vi "fix custom device xml.vi"(8 "error in (no error)":errorcluster, 10 "new xml path":path, 11 "CD name":string) -> (0 "error out":errorcluster)   [LabVIEW 2014, in "CD model script.lvlib"]
uses:
  CD model script.lvlib
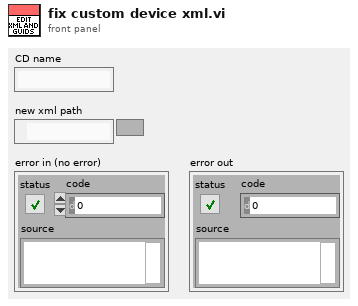
[diagram p1: front panel]
types:
  T1 = enum16{"open", "replace", "create", "open or create", "replace or create", "replace or create with confirmation"}
  T2 = typedef "CD model script.lvlib/CD Wizard - Extra Page Name and GUID.ctl" = cluster{"Page Name":string, "Page GUID":string}
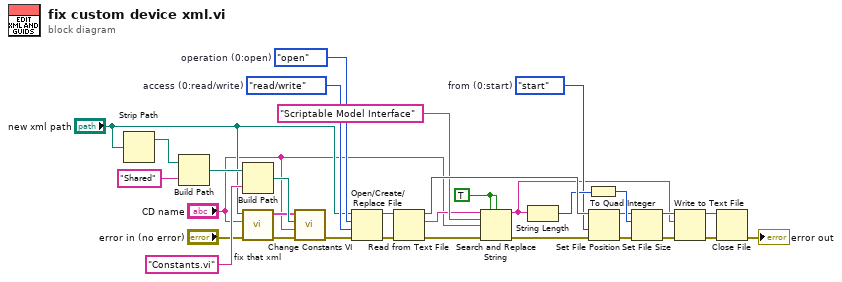
[diagram p0: block diagram]
diagram:
  w28 = enum16{"start", "end", "current"}."start"  # from (0:start)
  w21 = TRUE ("replace all? (F)")
  w17 = T1."open"  # operation (0:open)
  w16 = enum16{"read/write", "read-only", "write-only"}."read/write"  # access (0:read/write)
  n1 = Strip Path(path="new xml path") -> (stripped path=w11:path)  [unwired: 1 out]
  n2 = Build Path(base path=w11, name or relative path="Shared") -> (appended path=w10:path)
  n3 = Build Path(base path=w10, name or relative path="Constants.vi") -> (appended path=w7:path)
  n4 = call "fix that xml.vi"("error in (no error)"="error in (no error)", "nw CD name"="CD name", "Path"="new xml path") -> ("error out"=w12:errorcluster, "Extra Pages"=w6:T2[])  [unwired: 7 in]
  n5 = call "Change Constants VI.vi"("error in (no error)"=w12, "new cd name"="CD name", "Constants.vi path"=w7, "Extra Pages"=w6) -> ("error out"=w5:errorcluster)  [unwired: 7 in]
  n6 = Open/Create/Replace File(file path (use dialog)="new xml path", error in=w5, operation (0:open)=w17, access (0:read/write)=w16) -> (refnum out=w14:refnum<file>, error out=w15:errorcluster)  [unwired: 3 out]
  n7 = Read from Text File(file (use dialog)=w14, error in=w15) -> (refnum out=w31:refnum<file>, text=w18:string, error out=w19:errorcluster)  [unwired: 3 out]
  n8 = Search and Replace String(replace all?=w21, case sensitive?=w21, input string=w18, search string="Scriptable Model Interface", replace string="CD name", error in=w19) -> (result string=w13:string, error out=w32:errorcluster)  [unwired: 2 in, 2 out]
  n9 = String Length(string=w13) -> (length=w29:i32)
  n10 = To Quad Integer(1:w29) -> (0:w30:i64)
  n11 = Set File Position(refnum=w31, from (0:start)=w28, error in=w32) -> (refnum out=w27:refnum<file>, error out=w26:errorcluster)  [unwired: 1 out]
  n12 = Set File Size(4:w26, 6:w30, 7:w27) -> (0:w24:errorcluster, 3:w25:refnum<file>)
  n13 = Write to Text File(file (use dialog)=w25, text=w13, error in=w24) -> (refnum out=w22:refnum<file>, error out=w23:errorcluster)  [unwired: 2 out]
  n14 = Close File(refnum=w22, error in=w23) -> (error out=→"error out":errorcluster)  [unwired: 1 out]
